vi "HAPS_LoadTable_SetBeam_Manual_BoardCast.vi"() -> ()   [LabVIEW 2023, in "HAPS.lvlib"]
uses:
  HAPS.lvlib
  set_ele.ctl
  HAPS_SerialPort.ctl
  HAPS_MCU_ELE_Func.ctl
  <vilib>/Utility/file.llb/Read Delimited Spreadsheet (string).vi
  R_S/R_S.lvlib
panel:
  in  "OFF 13~15":bool
  in  "Init?":bool=TRUE
  in  "set_ele":T1={"ch"=0, "chain_id"=0, "group"=0, "array_id"=0, "ele_phase"=0, "ele_gain"=35, "com_gain"=17, "pd_range"=0}
  in  "file path (dialog if empty)":path=path "D:/_Project/_Code/LabVIEW/_CLC_Gen4/CLC_LV2023/CLC_Cali/Log/HAPS/Preset.csv"
  in  "VISA resource name":refnum<visa-resource-name>="COM1"
  out "Remaining quantity":i32
  out "ele phase":i32
  out "ele gain":i32
  out "channel":i32
  out "chain ID":i32
  out "group":i32
  out "array id":i32
  # "HAPS 24x24 Setting\nManual In-Phase_One"
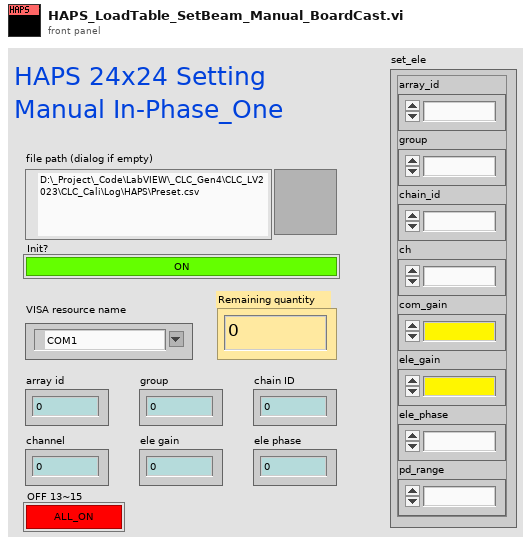
[diagram p1: front panel]
types:
  T1 = typedef "HAPS.lvlib/set_ele.ctl" = cluster{"ch":i32, "chain_id":i32, "group":i32, "array_id":i32, "ele_phase":i32, "ele_gain":i32, "com_gain":i32, "pd_range":i32}
  T2 = typedef "HAPS.lvlib/HAPS_MCU_ELE_Func.ctl" = enum16{"array_init", "set_com_gain", "set_ch_gain_phase", "set_pd_range", "get_preamp_temp", "get_bfic_temp", "get_tx_pd", "ch_on", "ch_on_2", "ch_ctrl_all", "array_ctrl_src"}
  T3 = typedef "HAPS.lvlib/HAPS_SerialPort.ctl" = enum16{"Init", "Close", "CMD", "Flush"}
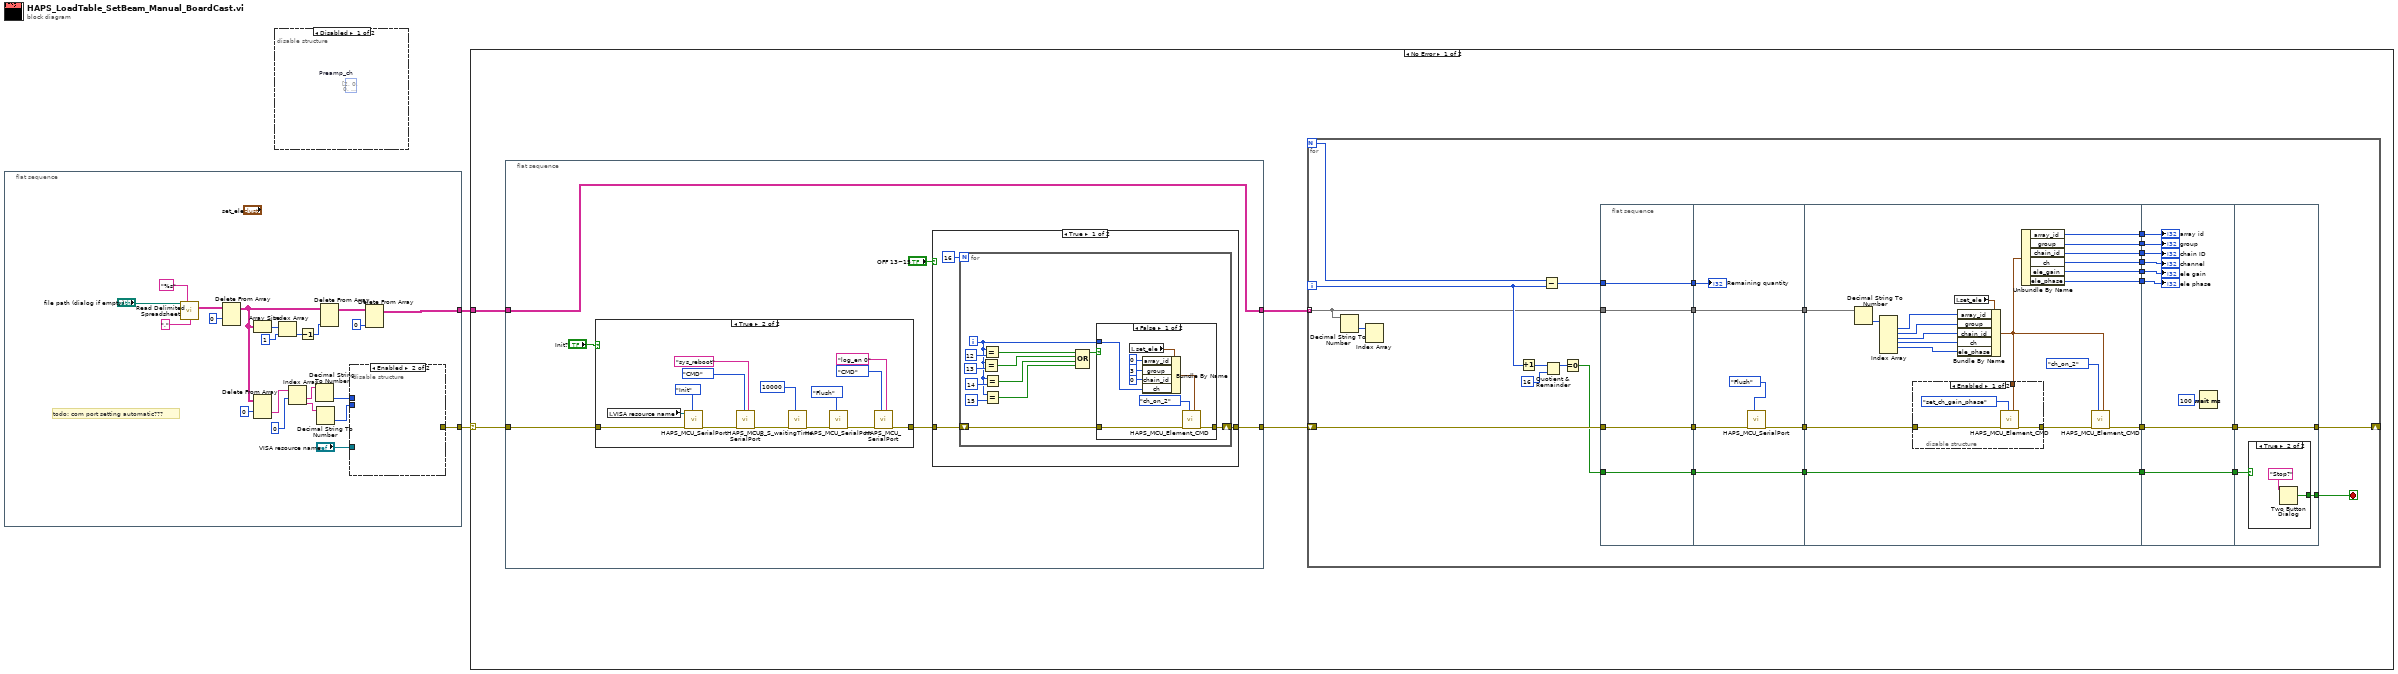
[diagram p0: block diagram]
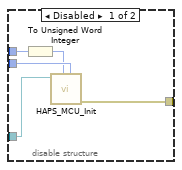
[diagram p2: hidden frame]
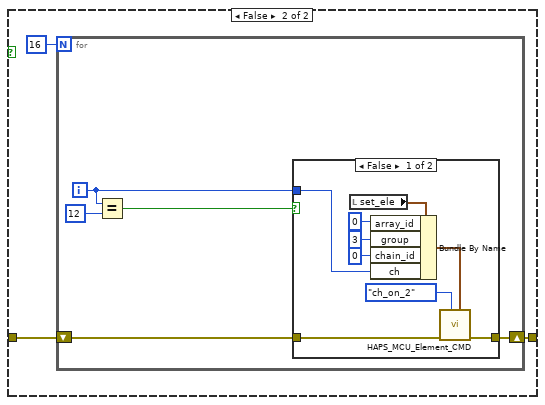
[diagram p5: hidden frame]
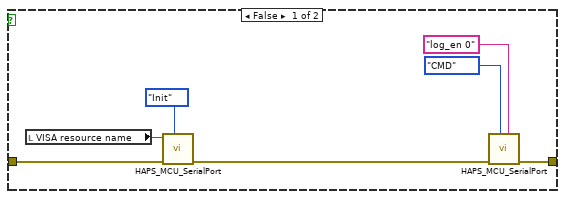
[diagram p7: hidden frame]
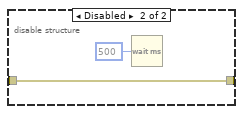
[diagram p8: hidden frame]
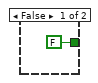
[diagram p9: hidden frame]
diagram:
  n1 = flat-sequence {
    tunnel: [w16] -> w2
    tunnel: [w3] -> w1
    frame #0 {
      # "todo: com port setting automatic???"
      n2 = call-poly <vilib>:"Read Delimited Spreadsheet.vi"("file path (dialog if empty)"="file path (dialog if empty)", "format (%s)"="%s" ("format (%.3f)"), "delimiter (\\t)"="," ("delimiter (\\t)")) -> ("all rows"=w22:string[][])  [unwired: 7 in, 5 out]
      n3 = Delete From Array(array=w22, index (row)=0) -> (array with subset deleted=w12:string[][])  [unwired: 2 in, 1 out]
      n4 = Array Size(array=w12) -> (size(s)=w20:i32[])
      n5 = Delete From Array(array=w12, index (row)=0) -> (deleted portion=w11:string[])  [unwired: 2 in, 1 out]
      n6 = Index Array(array=w20, index=1) -> (element=w17:i32)
      n7 = Index Array(array=w11, index #1=0 ("index")) -> (element #1=w10:string, element #2=w9:string)  [unwired: 1 in]
      n8 = Decrement(x=w17) -> (x-1=w19:i32)
      n9 = Decimal String To Number(string=w10) -> (number=w6:i32)  [unwired: 2 in, 1 out]
      n10 = Decimal String To Number(string=w9) -> (number=w5:i32)  [unwired: 2 in, 1 out]
      n11 = Delete From Array(array=w12, index (col)=w19) -> (array with subset deleted=w15:string[][])  [unwired: 2 in, 1 out]
      n12 = disable-structure shown="Enabled" {
        disable-tunnel: [w29 _] -> w16
        disable-tunnel: w6 -> [w28 _]
        disable-tunnel: w5 -> [w27 _]
        disable-tunnel: "VISA resource name" -> [w26 _]
        frame Disabled {
          n13 = To Unsigned Word Integer(number=w28) -> (unsigned 16bit integer=w25:u16)
          n14 = call "HAPS_MCU_Init.vi"("array_id"=w27, "Tx/Rx"=w25, "VISA resource name"=w26) -> ("error out"=w29:errorcluster)  [unwired: 8 in]
        }
        frame Enabled {
        }
      }
      n15 = Delete From Array(array=w15, index (col)=0 ("index (row)")) -> (array with subset deleted=w3:string[][])  [unwired: 2 in, 1 out]
    }
  }
  n16 = disable-structure shown="Disabled" {
    frame Disabled {
      (unwired) i32[][] [[2, 0, 0, 8, 8, 10, 11, 9, 9, 1, 1, 3], [3, 1, 1, 9, 9, 11, 13, 15, 15, 7, 7, 5], [5, 7, 7, 15, 15, 13, 14, 14, 6, 6, 4, 12]]  # Preamp_ch
    }
    frame Enabled {
    }
  }
  n17 = case shown="No Error" w2 {
    selector: w2 -> [w31 _]
    tunnel: w1 -> [w33 _]
    frame No Error {
      n18 = flat-sequence {
        tunnel: w33 -> [w39]
        tunnel: [w39] -> w32
        tunnel: w31 -> [w37]
        tunnel: [w38] -> w30
        frame #0 {
          n19 = case shown="True" "Init?" {
            tunnel: w37 -> [w87 w101]
            tunnel: [w85 w99] -> w36
            frame False {
              n20 = local read "VISA resource name"() -> (w83:refnum<visa-resource-name>)
              n21 = call "HAPS_MCU_SerialPort.vi"("HAPS_SerialPort_Func"=HAPS_SerialPort."Init", "error in"=w87, "VISA resource name"=w83) -> ("error out"=w84:errorcluster)  [unwired: 6 in, 2 out]
              n22 = call "HAPS_MCU_SerialPort.vi"("Command"="log_en 0", "HAPS_SerialPort_Func"=enum16{"Init", "Close", "CMD"}."CMD" ("HAPS_SerialPort"), "error in"=w84) -> ("error out"=w85:errorcluster)  [unwired: 6 in, 2 out]
            }
            frame True {
              n23 = local read "VISA resource name"() -> (w90:refnum<visa-resource-name>)
              n24 = call "HAPS_MCU_SerialPort.vi"("HAPS_SerialPort_Func"=HAPS_SerialPort."Init", "error in"=w101, "VISA resource name"=w90) -> ("error out"=w96:errorcluster)  [unwired: 6 in, 2 out]
              n25 = call "HAPS_MCU_SerialPort.vi"("Command"="sys_reboot", "HAPS_SerialPort_Func"=enum16{"Init", "Close", "CMD"}."CMD" ("HAPS_SerialPort"), "error in"=w96) -> ("error out"=w95:errorcluster)  [unwired: 6 in, 2 out]
              n26 = call "R_S_waitingTime.vi"("Waiting Time(ms)"=u32 10000, "error in"=w95) -> ("error out"=w93:errorcluster)  [unwired: 9 in]
              n27 = call "HAPS_MCU_SerialPort.vi"("HAPS_SerialPort_Func"=HAPS_SerialPort."Flush", "error in"=w93) -> ("error out"=w91:errorcluster)  [unwired: 7 in, 2 out]
              n28 = call "HAPS_MCU_SerialPort.vi"("Command"="log_en 0", "HAPS_SerialPort_Func"=enum16{"Init", "Close", "CMD"}."CMD" ("HAPS_SerialPort"), "error in"=w91) -> ("error out"=w99:errorcluster)  [unwired: 6 in, 2 out]
            }
          }
          n29 = case shown="True" "OFF 13~15" {
            tunnel: [w41 w66] -> w38
            tunnel: w36 -> [w40 w65]
            frame True {
              n30 = for {
                N: 16 -> [_]
                shift-right: [w53] -> w41
                shift-left: w40 -> [w54]
                i -> [w44]
                n31 = Equal?(x=w44, y=13) -> (x = y?=w48:bool)
                n32 = Equal?(x=w44, y=12) -> (x = y?=w52:bool)
                n33 = Equal?(x=w44, y=14) -> (x = y?=w46:bool)
                n34 = Equal?(x=w44, y=15) -> (x = y?=w43:bool)
                n35 = Compound Arithmetic op=OR(w52, w48, w46, w43) -> (w49:bool)
                n36 = case shown="False" w49 {
                  tunnel: w54 -> [w57 w64]
                  tunnel: [w56 w64] -> w53
                  tunnel: w44 -> [w55 _]
                  frame False {
                    n37 = local read "set_ele"() -> (w59:T1)
                    n38 = Bundle By Name(cluster=w59, "array_id"=0, "group"=3, "chain_id"=0, "ch"=w55) -> (w60:T1)
                    n39 = call "HAPS_MCU_Element_CMD.vi"("set_ele"=w60, "HAPS_MCU_ELE_Func."=HAPS_MCU_ELE_Func."ch_on_2", "error in"=w57) -> ("error out"=w56:errorcluster)  [unwired: 7 in, 1 out]
                  }
                  frame True {
                  }
                }
              }
            }
            frame False {
              n40 = for {
                N: 16 -> [_]
                shift-right: [w71] -> w66
                shift-left: w65 -> [w72]
                i -> [w69]
                n41 = Equal?(x=w69, y=12) -> (x = y?=w68:bool)
                n42 = case shown="False" w68 {
                  tunnel: w72 -> [w75 w82]
                  tunnel: [w74 w82] -> w71
                  tunnel: w69 -> [w73 _]
                  frame False {
                    n43 = local read "set_ele"() -> (w77:T1)
                    n44 = Bundle By Name(cluster=w77, "array_id"=0, "group"=3, "chain_id"=0, "ch"=w73) -> (w78:T1)
                    n45 = call "HAPS_MCU_Element_CMD.vi"("set_ele"=w78, "HAPS_MCU_ELE_Func."=HAPS_MCU_ELE_Func."ch_on_2", "error in"=w75) -> ("error out"=w74:errorcluster)  [unwired: 7 in, 1 out]
                  }
                  frame True {
                  }
                }
              }
            }
          }
        }
      }
      n46 = for {
        N -> [w130]
        tunnel: w32 -> [w127] mode=indexing
        shift-right: [w132] -> _
        shift-left: w30 -> [w131]
        i -> [w129]
        stop <- w104 stop-if-true
        n47 = Decimal String To Number(string=w127) -> (number=w128:i32[])  [unwired: 2 in, 1 out]
        n48 = Index Array(array=w128) -> ()  [unwired: 2 in, 2 out]
        n49 = Increment(x=w129) -> (x+1=w108:i32)
        n50 = Subtract(x=w130, y=w129) -> (x-y=w109:i32)
        n51 = Quotient & Remainder(x=w108, y=16) -> (x-y*floor(x/y)=w106:i32)  [unwired: 1 out]
        n52 = Equal To 0?(x=w106) -> (x = 0?=w105:bool)
        n53 = flat-sequence {
          tunnel: w109 -> [w134]
          tunnel: w131 -> [w135]
          tunnel: w127 -> [w136]
          tunnel: [w136] -> w126
          tunnel: [w135] -> w125
          tunnel: [w134] -> w124
          tunnel: w105 -> [w133]
          tunnel: [w133] -> w123
          tunnel: [w141] -> w122
          tunnel: [w139] -> w121
          tunnel: w126 -> [w141]
          tunnel: w125 -> [w138]
          tunnel: w124 -> [w142]
          tunnel: w123 -> [w137]
          tunnel: [w137] -> w120
          tunnel: w122 -> [w162]
          tunnel: w121 -> [w160]
          tunnel: [w147] -> w119
          tunnel: [w156] -> w118
          tunnel: [w155] -> w117
          tunnel: [w154] -> w116
          tunnel: [w153] -> w115
          tunnel: [w152] -> w114
          tunnel: [w151] -> w113
          tunnel: w120 -> [w143]
          tunnel: [w143] -> w112
          tunnel: w119 -> [w177]
          tunnel: w118 -> [w176]
          tunnel: w117 -> [w175]
          tunnel: w116 -> [w174]
          tunnel: w115 -> [w173]
          tunnel: w114 -> [w172]
          tunnel: w113 -> [w171]
          tunnel: [w177] -> w111
          tunnel: w112 -> [w169]
          tunnel: [w169] -> w110
          tunnel: [w180] -> w132
          tunnel: w111 -> [w180]
          tunnel: w110 -> [w179]
          tunnel: [w178] -> w104
          frame #0 {
          }
          frame #1 {
            n54 = call "HAPS_MCU_SerialPort.vi"("HAPS_SerialPort_Func"=HAPS_SerialPort."Flush", "error in"=w138) -> ("error out"=w139:errorcluster)  [unwired: 7 in, 2 out]
            "Remaining quantity" <- w142
          }
          frame #2 {
            n55 = Decimal String To Number(string=w162) -> (number=w161:i32[])  [unwired: 2 in, 1 out]
            n56 = Index Array(array=w161) -> (element #1=w159:i32, element #2=w150:i32, element #3=w149:i32, element #4=w158:i32, element #5=w157:i32)  [unwired: 6 in, 1 out]
            n57 = local read "set_ele"() -> (w144:T1)
            n58 = Bundle By Name(cluster=w144, "array_id"=w159, "group"=w150, "chain_id"=w149, "ch"=w158, "ele_phase"=w157) -> (w145:T1)
            n59 = disable-structure shown="Enabled" {
              disable-tunnel: [w166 w168] -> w148
              disable-tunnel: w160 -> [w165 w168]
              disable-tunnel: w145 -> [w163 _]
              frame Enabled {
                n60 = call "HAPS_MCU_Element_CMD.vi"("set_ele"=w163, "HAPS_MCU_ELE_Func."=HAPS_MCU_ELE_Func."set_ch_gain_phase", "error in"=w165) -> ("error out"=w166:errorcluster)  [unwired: 7 in, 1 out]
              }
              frame Disabled {
                n61 = Wait (ms)(milliseconds to wait=u32 500) -> ()  [unwired: 1 out]
              }
            }
            n62 = Unbundle By Name(w145) -> ("array_id"=w156:i32, "group"=w155:i32, "chain_id"=w154:i32, "ch"=w153:i32, "ele_gain"=w152:i32, "ele_phase"=w151:i32)
            n63 = call "HAPS_MCU_Element_CMD.vi"("set_ele"=w145, "HAPS_MCU_ELE_Func."=HAPS_MCU_ELE_Func."ch_on_2", "error in"=w148) -> ("error out"=w147:errorcluster)  [unwired: 7 in, 1 out]
          }
          frame #3 {
            n64 = Wait (ms)(milliseconds to wait=u32 100) -> ()  [unwired: 1 out]
            "group" <- w175
            "chain ID" <- w174
            "channel" <- w173
            "ele gain" <- w172
            "ele phase" <- w171
            "array id" <- w176
          }
          frame #4 {
            n65 = case shown="True" w179 {
              tunnel: [FALSE ("T button?") w182] -> w178
              frame False {
              }
              frame True {
                n66 = Two Button Dialog(message="Stop?") -> (T button?=w182:bool)  [unwired: 2 in]
              }
            }
          }
        }
      }
    }
    frame Error {
    }
  }
